vi "Create.vi"(8 "error in (no error)":errorcluster, 11 "TEST in":refnum<class "TEST1.lvclass">) -> (0 "error out":errorcluster, 3 "TEST out":refnum<class "TEST1.lvclass">)   [LabVIEW 2021, in "TEST1.lvclass"]
uses:
  TEST1.lvclass
  D:/my_projects/projects/Algorithms/Labview/21/Master CR/Master CR.lvclass
  Data Model/ICPCON ET7000 Data Model/TEST/TEST Data Model.lvclass
  D:/my_projects/projects/Algorithms/Labview/21/Modbus_v121c/Data Model/Device Data Model.lvclass
  Master CR.lvclass/Master CR.ctl
  TCP/TCP.lvclass
  TEST1.lvclass/TEST1.ctl
  Master CR.lvclass
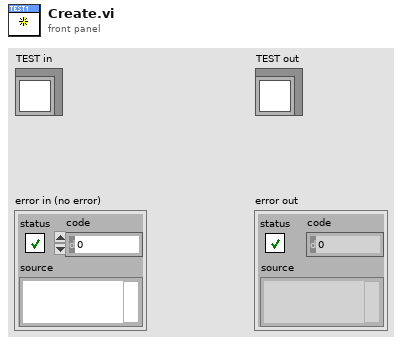
[diagram p1: front panel]
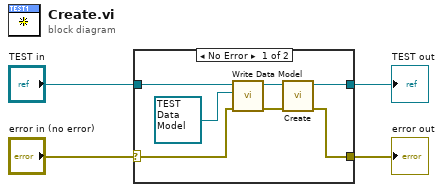
[diagram p0: block diagram]
diagram:
  n1 = case shown="No Error" "error in (no error)" {
    selector: "error in (no error)" -> [w5 w12]
    tunnel: [w9 w12] -> w2
    tunnel: [w10 w13] -> w3
    tunnel: "TEST in" -> [w11 w13]
    frame No Error {
      n2 = call "Write Data Model.vi"("error in (no error)"=w5, "Data Model"=refnum<class "TEST Data Model.lvclass"> refnum ("Modbus API:Device Data Model"), "Master CR in"=w11) -> ("error out"=w7:errorcluster, "Master CR out"=w8:refnum<class "TEST1.lvclass">)  [unwired: 7 in]
      n3 = call-parent "Create.vi"("error in (no error)"=w7, "TCP in"=w8) -> ("error out"=w9:errorcluster, "TCP out"=w10:refnum<class "TEST1.lvclass">)  [unwired: 8 in]
    }
    frame Error {
    }
  }
  "error out" <- w2
  "TEST out" <- w3
